vi "get outgoing Interaction Information element by name.vi"(10 "name":string, 11 "interaction_attribute_type":T1) -> (1 "found":bool, 3 "element out":dbl)   [LabVIEW 2019, in "HLA Custom Device Engine.lvlib"]
uses:
  HLA Custom Device Engine.lvlib
  _typedefs/interaction_info_outgoing_type.ctl
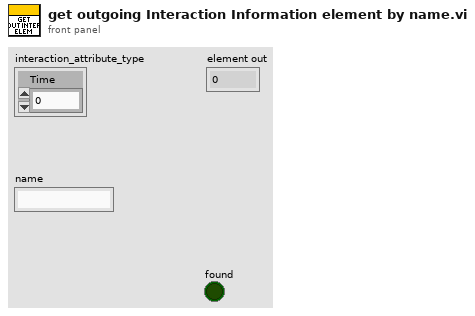
[diagram p1: front panel]
types:
  T1 = typedef "HLA Custom Device Engine.lvlib/interaction_info_outgoing_type.ctl" = cluster{"Time":dbl}
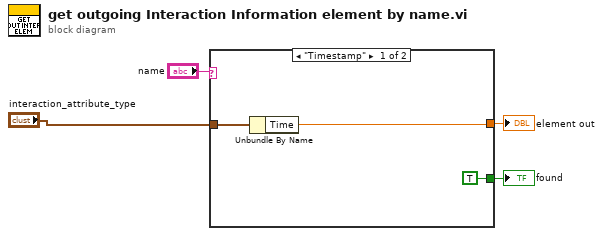
[diagram p0: block diagram]
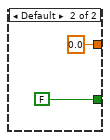
[diagram p2: hidden frame]
diagram:
  n1 = case shown="\"Timestamp\"" "name" {
    tunnel: "interaction_attribute_type" -> [w6 _]
    tunnel: [w7 0.0] -> w2
    tunnel: [TRUE FALSE] -> w1
    frame "Timestamp" {
      n2 = Unbundle By Name(w6) -> ("Time"=w7:dbl)
    }
    frame Default {
    }
  }
  "element out" <- w2
  "found" <- w1
